vi "01_Splitter_Panes_solution.vi"() -> ()   [LabVIEW 2020]
panel:
  in  "Arrow Right":bool
  in  "Arrow Left":bool
  in  "Close":bool
  in  "Stop":bool
  in  "File":bool
  in  "Settings":bool
  in  "Listbox":i32(listbox)
  out "Waveform Graph":dbl[](graph)
  out "StatusBarLeft":string
  out "StatusBarCenter":string
  out "StatusBarRight":string
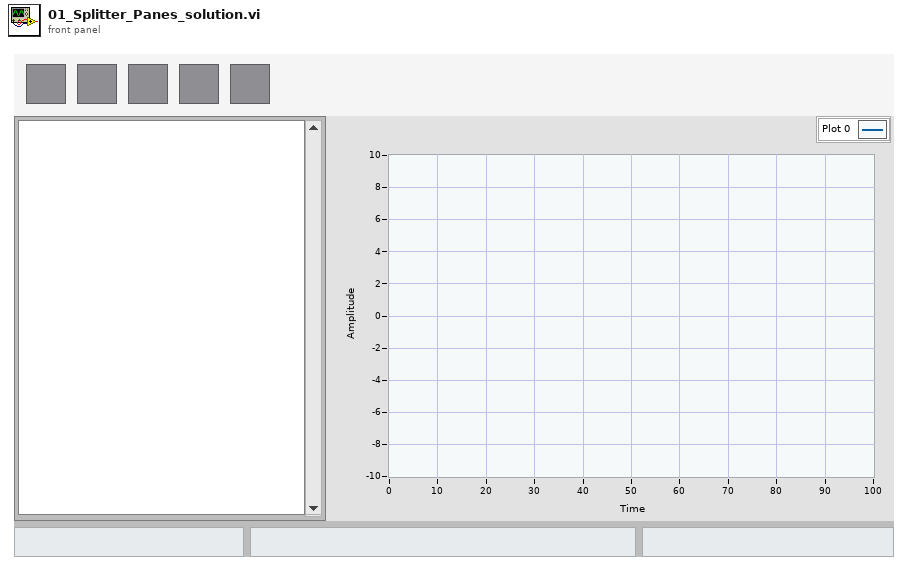
[diagram p1: front panel]
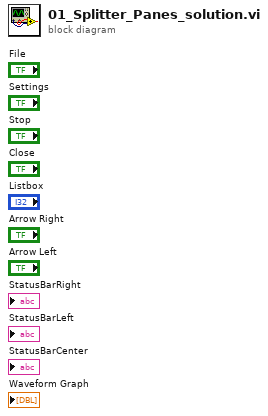
[diagram p0: block diagram]
diagram:
